vi "SQL Get DB Schema.vi"() -> ()   [LabVIEW 2009]
panel:
  out "return code":i32
  out "Tables":T1(array[cluster])
  out "error out":errorcluster
  in  "error in (no error)":errorcluster
  out "Table Name":string[](array[string])
  in  "Database Name":string
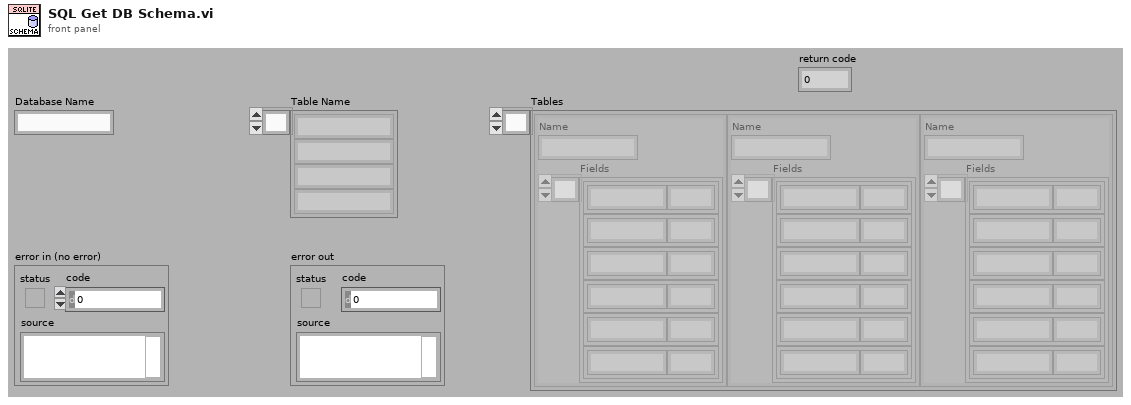
[diagram p1: front panel]
types:
  T1 = cluster{"Name":string, "Fields":cluster{"Name":string, "Type":string}[]}[]
  T2 = cluster{string, cluster{"Name":string, "Type":string}[]}
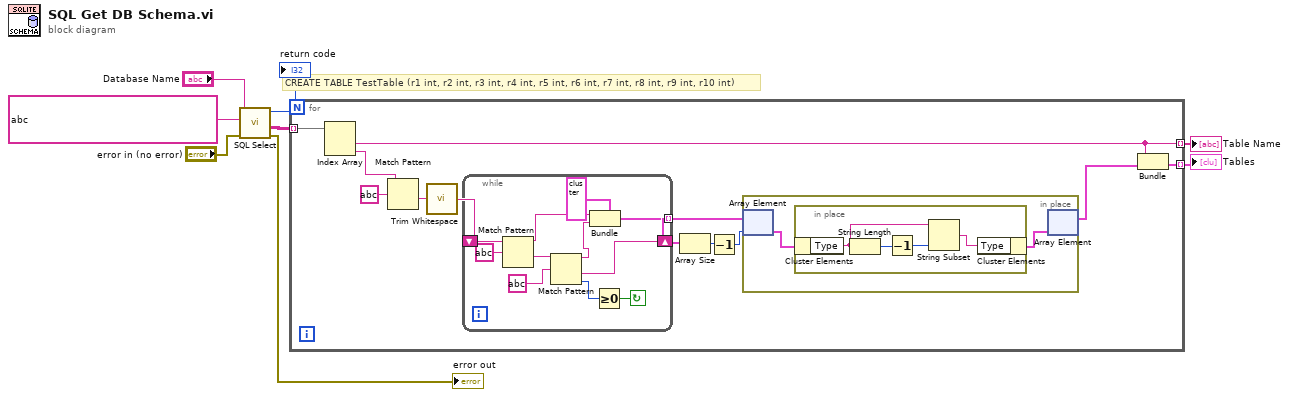
[diagram p0: block diagram]
diagram:
  # "CREATE TABLE TestTable (r1 int, r2 int, r3 int, r4 int, r5 int, r6 int, r7 int, r8 int, r9 int, r10 int)"
  n1 = call "SQL Select.vi"("error in (no error)"="error in (no error)", "Select Statement"=string ?, "Database Name"="Database Name") -> ("error out"=→"error out":errorcluster, "Select Result"=w5:string[][], "return code"=→"return code":i32)  [unwired: 5 in, 1 out]
  n2 = for {
    tunnel: w5 -> [w19] mode=indexing
    tunnel: [w16] -> w4 mode=indexing
    tunnel: [w15] -> w3 mode=indexing
    n3 = Index Array(array=w19) -> (element #1=w16:string, element #2=w18:string)  [unwired: 2 in]
    n4 = Match Pattern(string=w18, regular expression=string ?) -> (after substring=w14:string)  [unwired: 1 in, 3 out]
    n5 = call <vilib>:"Trim Whitespace.vi"("string"=w14) -> ("trimmed string"=w13:string)  [unwired: 1 in]
    n6 = while {
      shift-right: [w30] -> _
      shift-left: w13 -> [w36]
      tunnel: [w27] -> w12 mode=indexing
      stop <- w31 continue-if-true
      n7 = Match Pattern(string=w36, regular expression=string ?) -> (before substring=w28:string, after substring=w34:string)  [unwired: 1 in, 2 out]
      n8 = Match Pattern(string=w34, regular expression=string ?) -> (before substring=w29:string, after substring=w30:string, offset past match=w32:i32)  [unwired: 1 in, 1 out]
      n9 = Bundle(cluster=cluster{"Name":string, "Type":string} ?, "Name"=w28, "Type"=w29) -> (w27:cluster{"Name":string, "Type":string})
      n10 = Greater Or Equal To 0?(x=w32) -> (x >= 0?=w31:bool)
    }
    n11 = Array Size(array=w12) -> (size(s)=w10:i32)
    n12 = Decrement(x=w10) -> (x-1=w9:i32)
    n13 = in-place {
      n14 = in-place-array #1(w12, w9) -> (w21:cluster{"Name":string, "Type":string})
      n15 = in-place {
        n16 = in-place-cluster #2(w21) -> ("Type"=w25:string)
        n17 = String Length(string=w25) -> (length=w23:i32)
        n18 = Decrement(x=w23) -> (x-1=w22:i32)
        n19 = String Subset(string=w25, length (rest)=w22) -> (substring=w24:string)  [unwired: 1 in]
        n20 = in-place-cluster #2("Type"=w24) -> (w20:cluster{"Name":string, "Type":string})
      }
      n21 = in-place-array #1(w20) -> (w11:cluster{"Name":string, "Type":string}[])  [unwired: 1 out]
    }
    n22 = Bundle(w16, w11) -> (w15:T2)  [unwired: 1 in]
  }
  "Table Name" <- w4
  "Tables" <- w3
